vi "PCF8591_AO.vi"(8 "error in (no error)":errorcluster, 11 "DAC (0-255)":u8) -> (0 "error out":errorcluster)   [LabVIEW 2014, in "QwaveSys RPi Training Library.lvlib"]
uses:
  <vilib>/Q-Wave Systems/QwaveSys RPi Package 2.0/Addons/QwaveSys RPi Training Library.lvlib
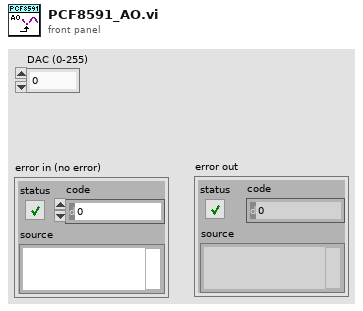
[diagram p1: front panel]
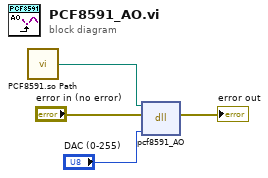
[diagram p0: block diagram]
diagram:
  n1 = call <vilib>:"PCF8591.so Path.vi"() -> ("PCF8591.so Path"=w2:path)  [unwired: 5 in]
  n2 = dll-call lib="pcf8591.so" fn="pcf8591_AO"(path in=w2, error in="error in (no error)", "dac"="DAC (0-255)") -> (error out=→"error out":errorcluster)  [unwired: 3 in, 1 out]
